vi "init Tx.vi"(10 "Tx UDP config":cluster{"Timeout":u16, "Local Port":u16}={"Timeout"=1, "Local Port"=1234}) -> (0 "error out":errorcluster, 3 "UDP Tx.lvclass":refnum<class "UDP Tx.lvclass">)   [LabVIEW 2012, in "UDP Tx.lvclass"]
uses:
  UDP Tx.lvclass
  UDP Tx.lvclass/UDP Tx.ctl
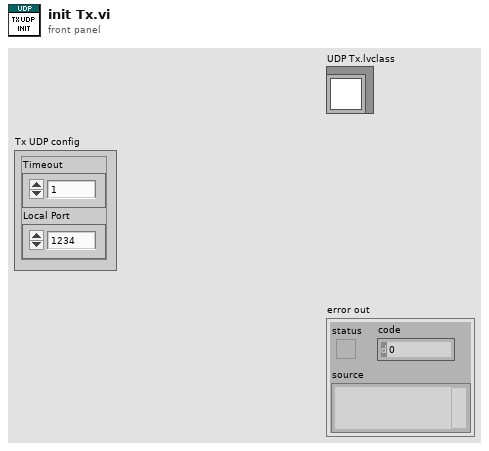
[diagram p1: front panel]
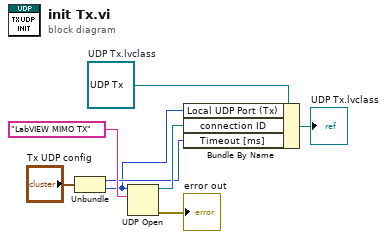
[diagram p0: block diagram]
diagram:
  w8 = refnum<class "UDP Tx.lvclass"> refnum  # UDP Tx.lvclass
  n1 = Unbundle("Tx UDP config") -> ("Timeout"=w3:u16, "Local Port"=w2:u16)
  n2 = UDP Open(10:"LabVIEW MIMO TX" ("service name"), 11:w2) -> (port=w5:refnum<k16>, 0:→"error out":errorcluster)  [unwired: 3 in, 1 out]
  n3 = Bundle By Name(cluster=w8, "Local UDP Port (Tx)"=w2, "connection ID"=w5, "Timeout [ms]"=w3) -> (→"UDP Tx.lvclass":refnum<class "UDP Tx.lvclass">)
